vi "Initialize Custom Device.vi"(8 "error in":errorcluster, 11 "custom device ref":T1=18446744073709551615 format="%.0x") -> (0 "error out":errorcluster, 3 "custom device ref out":T1 format="%.0x")   [LabVIEW 2020, in "Communication Bus Template Scripting.lvlib"]
uses:
  Communication Bus Template Scripting.lvlib
  <vilib>/NI VeriStand/Custom Device API/Custom Device Item Ref.ctl
  <vilib>/NI VeriStand/Custom Device API/Custom Device API.lvlib
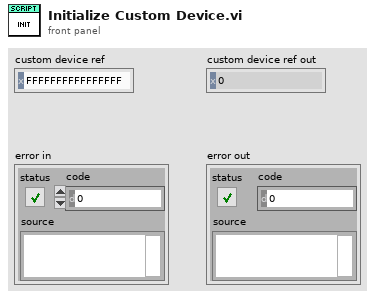
[diagram p1: front panel]
types:
  T1 = typedef "Custom Device API.lvlib/Custom Device Item Ref.ctl" = u64
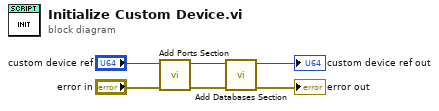
[diagram p0: block diagram]
diagram:
  n1 = call "Add Ports Section.vi"("error in"="error in", "Custom device Ref"="custom device ref") -> ("error out"=w5:errorcluster, "Custom device Ref out"=w6:T1)  [unwired: 8 in]
  n2 = call "Add Databases Section.vi"("error in"=w5, "Custom device Ref"=w6) -> ("error out"=→"error out":errorcluster, "Custom device Ref out"=→"custom device ref out":T1)  [unwired: 8 in]
